vi "PH_PPMA_PowerUnit.set  prdc period.vi"(0 "i ref in":refnum<vi>, 2 "Waiting Time (s)":i32, 5 "error in (no error)":errorcluster) -> (14 "i ref out":refnum<vi>, 19 "error out":errorcluster)   [LabVIEW 2014, in "PH_PPMA_PowerUnit.lvlib"]
doc: "This VI sets the periodic interval. This depends on the remaining waiting time (if this remaining time is shorter than 3Xdefault prdc interval, the periodic interval is set to 1s; otherwise the default value is chosen)."
uses:
  PH_PPMA_PowerUnit.lvlib
  CS_Core/BaseProcess/BaseProcess.lvlib
  CS_Core/CSSystem/CSSystemLib/CSSystemLib.lvlib
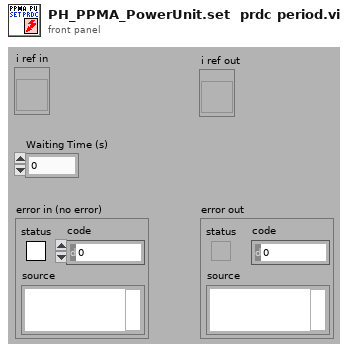
[diagram p1: front panel]
types:
  T1 = typedef "PH_PPMA_PowerUnit.lvlib/PH_PPMA_PowerUnit.i attribute.ctl" = cluster{"GUI Refs":cluster{"Rods":refnum<vi>, "Ignitron":refnum<vi>, "Rossrelais":refnum<vi>, "Set Voltage":refnum<vi>, "PSU":refnum<vi>, "EOC":refnum<vi>, "Trigger":refnum<vi>}, "Rods":T2, "PSU":T4, "Ross Relais":T5, "Ignitron":T6, "Trigger":cluster{"State Device":T3, "linked?":bool}, "Timing Settings":cluster{"Prdc Fast?":bool, "Default Value Periodic Interval":i32, "Mercury on since":dbl, "Warm up Time Mercury [s]":dbl}, "Set Voltage [V]":dbl}
  T2 = typedef "PH_PPMA_PowerUnit.lvlib/PH_PPMA_PowerUnit.Rods Attributes.ctl" = cluster{"Instancename":string, "Device Status":T3, "linked?":bool}
  T3 = typedef "PH_StatusHandler.lvlib/PH_StatusHandler.Status.ctl" = i16
  T4 = typedef "PH_PP_Common.lvlib/PH_PP_Common.PSU Attributes.ctl" = cluster{"lower limit [V]":dbl, "upper limit [V]":dbl, "Voltage set":bool, "State Device":T3, "linked?":bool}
  T5 = typedef "PH_PP_Common.lvlib/PH_PP_Common.Ross Relais Attributes.ctl" = cluster{"State Device":T3, "linked?":bool}
  T6 = typedef "PH_PP_Common.lvlib/PH_PP_Common.Ignitron Attributes.ctl" = cluster{"State Device":T3, "linked?":bool}
  T7 = enum16{"simple", "synchronous", "asynchronous", "notification"}
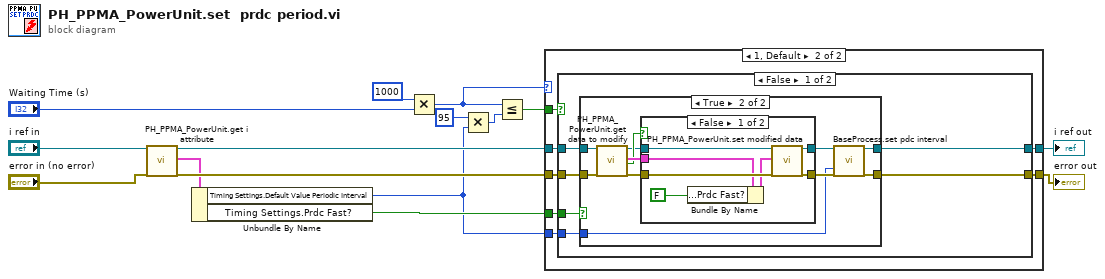
[diagram p0: block diagram]
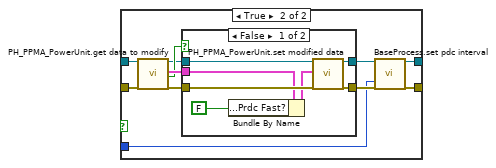
[diagram p3: hidden frame]
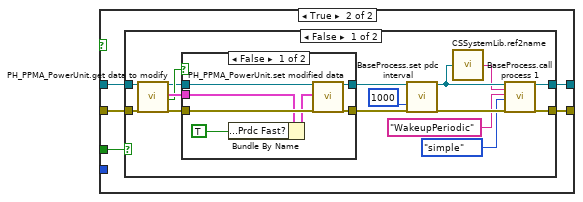
[diagram p7: hidden frame]
diagram:
  n1 = call "PH_PPMA_PowerUnit.get i attribute.vi"("i ref in"="i ref in", "error in (no error)"="error in (no error)") -> ("i ref out"=w12:refnum<vi>, "i attribute"=w7:T1, "error out"=w13:errorcluster)  [unwired: 15 in]
  n2 = Unbundle By Name(w7) -> ("Timing Settings.Default Value Periodic Interval"=w2:i32, "Timing Settings.Prdc Fast?"=w4:bool)
  n3 = Multiply(x=1000, y="Waiting Time (s)") -> (x*y=w1:i32)
  n4 = Multiply(x=95, y=w2) -> (x*y=w10:i32)
  n5 = Less Or Equal?(x=w1, y=w10) -> (x <= y?=w3:bool)
  n6 = case shown="1, Default" w1 {
    tunnel: [w18 w50] -> w15
    tunnel: [w19 w49] -> w14
    tunnel: w13 -> [w20 w48]
    tunnel: w12 -> [w21 w47]
    tunnel: w4 -> [w16 w46]
    tunnel: w3 -> [_ w45]
    tunnel: w2 -> [w17 w44]
    frame 0 {
      n7 = case shown="False" w16 {
        tunnel: w21 -> [w23 w28]
        tunnel: w20 -> [w22 w27]
        tunnel: [w23 w26] -> w19
        tunnel: [w22 w25] -> w18
        tunnel: w17 -> [_ w24]
        frame False {
        }
        frame True {
          n8 = call "PH_PPMA_PowerUnit.get data to modify.vi"("i ref in"=w28, "error in (no error)"=w27) -> ("i ref out"=w30:refnum<vi>, "i attribute"=w32:T1, "timed out"=w31:bool, "error out"=w29:errorcluster)  [unwired: 14 in]
          n9 = case shown="False" w31 {
            tunnel: w29 -> [w41 w42]
            tunnel: w30 -> [w40 w43]
            tunnel: [w39 w43] -> w33
            tunnel: [w38 w42] -> w34
            tunnel: w32 -> [w37 _]
            frame False {
              n10 = Bundle By Name(cluster=w37, "Timing Settings.Prdc Fast?"=FALSE) -> (w36:T1)
              n11 = call "PH_PPMA_PowerUnit.set modified data.vi"("i ref in"=w40, "i attribute"=w36, "error in (no error)"=w41) -> ("i ref out"=w39:refnum<vi>, "error out"=w38:errorcluster)  [unwired: 15 in]
            }
            frame True {
            }
          }
          n12 = call "BaseProcess.set pdc interval.vi"("i ref in"=w33, "PeriodicInterval [ms]"=w24, "error in (no error)"=w34) -> ("i ref out"=w26:refnum<vi>, "error out"=w25:errorcluster)  [unwired: 14 in, 1 out]
        }
      }
    }
    frame 1, Default {
      n13 = case shown="False" w45 {
        tunnel: [w53 w83] -> w50
        tunnel: [w54 w82] -> w49
        tunnel: w48 -> [w55 w81]
        tunnel: w47 -> [w56 w80]
        tunnel: w46 -> [w51 w79]
        tunnel: w44 -> [w52 _]
        frame False {
          n14 = case shown="True" w51 {
            tunnel: w56 -> [w58 w63]
            tunnel: w55 -> [w57 w62]
            tunnel: [w58 w61] -> w54
            tunnel: [w57 w60] -> w53
            tunnel: w52 -> [_ w59]
            frame False {
            }
            frame True {
              n15 = call "PH_PPMA_PowerUnit.get data to modify.vi"("i ref in"=w63, "error in (no error)"=w62) -> ("i ref out"=w65:refnum<vi>, "i attribute"=w67:T1, "timed out"=w66:bool, "error out"=w64:errorcluster)  [unwired: 14 in]
              n16 = case shown="False" w66 {
                tunnel: w64 -> [w76 w77]
                tunnel: w65 -> [w75 w78]
                tunnel: [w74 w78] -> w68
                tunnel: [w73 w77] -> w69
                tunnel: w67 -> [w72 _]
                frame False {
                  n17 = Bundle By Name(cluster=w72, "Timing Settings.Prdc Fast?"=FALSE) -> (w71:T1)
                  n18 = call "PH_PPMA_PowerUnit.set modified data.vi"("i ref in"=w75, "i attribute"=w71, "error in (no error)"=w76) -> ("i ref out"=w74:refnum<vi>, "error out"=w73:errorcluster)  [unwired: 15 in]
                }
                frame True {
                }
              }
              n19 = call "BaseProcess.set pdc interval.vi"("i ref in"=w68, "PeriodicInterval [ms]"=w59, "error in (no error)"=w69) -> ("i ref out"=w61:refnum<vi>, "error out"=w60:errorcluster)  [unwired: 14 in, 1 out]
            }
          }
        }
        frame True {
          n20 = case shown="False" w79 {
            tunnel: [w98 w109] -> w83
            tunnel: [w96 w110] -> w82
            tunnel: w81 -> [w87 w109]
            tunnel: w80 -> [w86 w110]
            frame False {
              n21 = call "PH_PPMA_PowerUnit.get data to modify.vi"("i ref in"=w86, "error in (no error)"=w87) -> ("i ref out"=w85:refnum<vi>, "i attribute"=w89:T1, "timed out"=w88:bool, "error out"=w84:errorcluster)  [unwired: 14 in]
              n22 = case shown="False" w88 {
                tunnel: w84 -> [w106 w107]
                tunnel: w85 -> [w105 w108]
                tunnel: [w104 w108] -> w97
                tunnel: [w103 w107] -> w99
                tunnel: w89 -> [w102 _]
                frame False {
                  n23 = Bundle By Name(cluster=w102, "Timing Settings.Prdc Fast?"=TRUE) -> (w101:T1)
                  n24 = call "PH_PPMA_PowerUnit.set modified data.vi"("i ref in"=w105, "i attribute"=w101, "error in (no error)"=w106) -> ("i ref out"=w104:refnum<vi>, "error out"=w103:errorcluster)  [unwired: 15 in]
                }
                frame True {
                }
              }
              n25 = call "BaseProcess.set pdc interval.vi"("i ref in"=w97, "PeriodicInterval [ms]"=1000 ("PeriodicInterval"), "error in (no error)"=w99) -> ("i ref out"=w94:refnum<vi>, "error out"=w95:errorcluster)  [unwired: 14 in, 1 out]
              n26 = call "CSSystemLib.ref2name.vi"("obj refnum"=w94) -> ("name"=w92:string)
              n27 = call "BaseProcess.call process 1.vi"("i ref in"=w94, "Object"=w92, "Selector"="WakeupPeriodic", "CallType"=T7."simple", "error in (no error)"=w95) -> ("i ref out"=w96:refnum<vi>, "error out"=w98:errorcluster)  [unwired: 12 in, 1 out]
            }
            frame True {
            }
          }
        }
      }
    }
  }
  "error out" <- w15
  "i ref out" <- w14
